vi "CSM - Read INI String.vi"(4 "Write If not found?(F)":bool, 5 "Section Name(\"\" as Default)":string, 7 "error in (no error)":errorcluster, 8 ">> Default Value >>":string, 9 "String in":string) -> (1 "error out":errorcluster, 2 "Key Found?":bool, 3 "String out":string)   [LabVIEW 2017, in "INI-Static-Variable-Support.lvlib"]
uses:
  INI-Static-Variable-Support.lvlib
  _fgv-oper.ctl
  global-csm-ini-db-change-flag.vi
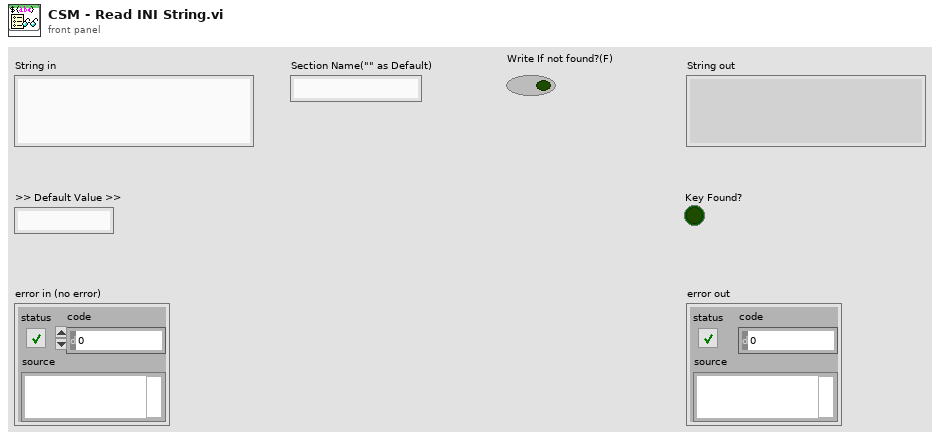
[diagram p1: front panel]
types:
  T1 = typedef "INI-Static-Variable-Support.lvlib/_fgv-oper.ctl" = enum16{"Read", "Write", "Sync", "Sessions", "List Keys", "Load", "List Files", "List Variables", "List Permanent Variables", "Mark Temp Variable as Permenent", "unload", "INIConfig(Memory)", "Reset", "Restore Variable Value"}
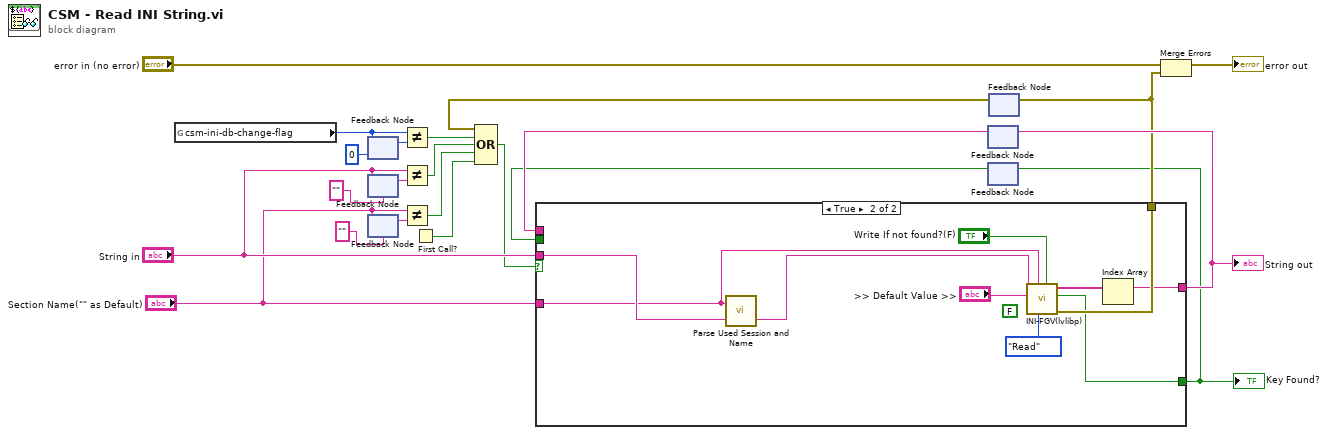
[diagram p0: block diagram]
diagram:
  n1 = global read "global-csm-ini-db-change-flag.vi" "csm-ini-db-change-flag"() -> (w20:u64)
  n2 = feedback #1(u64 0 ("csm-ini-db-change-flag")) -> (w19:u64)
  n3 = feedback-in #1(w20) -> ()
  n4 = feedback #2("") -> (w17:string)
  n5 = feedback-in #2("String in") -> ()
  n6 = feedback #3("") -> (w16:string)
  n7 = feedback-in #3("Section Name(\"\" as Default)") -> ()
  n8 = Not Equal?(x=w20, y=w19) -> (x != y?=w18:bool)
  n9 = Not Equal?(x="String in", y=w17) -> (x != y?=w13:bool)
  n10 = Not Equal?(x="Section Name(\"\" as Default)", y=w16) -> (x != y?=w12:bool)
  n11 = First Call?() -> (First Call?: T/F=w1:bool)
  n12 = feedback #4() -> (w10:string)  [unwired: 1 in]
  n13 = feedback #5() -> (w7:bool)  [unwired: 1 in]
  n14 = feedback #6() -> (w6:errorcluster)  [unwired: 1 in]
  n15 = Compound Arithmetic op=OR(w6, w18, w13, w12, w1) -> (w5:bool)
  n16 = case shown="True" w5 {
    tunnel: [_ w32] -> w9
    tunnel: [w24 w29] -> w11
    tunnel: [w23 w30] -> w8
    tunnel: "String in" -> [_ w27]
    tunnel: "Section Name(\"\" as Default)" -> [_ w25]
    tunnel: w10 -> [w24 _]
    tunnel: w7 -> [w23 _]
    frame False {
    }
    frame True {
      (unwired) FALSE ("Raw String? (F)")
      n17 = call "Parse Used Session and Name.vi"("name"=w27, "Section Name(\"\" as Default)"=w25) -> ("used name"=w26:string)  [unwired: 1 in]
      n18 = call "INI-FGV(lvlibp).vi"("Write If not found?"="Write If not found?(F)", "Enum"=_fgv-oper."Read", "Prefered Section"=w25, ">> Default Value >>"=">> Default Value >>", ">> Variable Name >>"=w26) -> ("error out"=w32:errorcluster, "Key?"=w30:bool, "Array"=w31:string[])  [unwired: 3 in, 1 out]
      n19 = Index Array(array=w31) -> (element=w29:string)  [unwired: 1 in]
    }
  }
  "String out" <- w11
  "Key Found?" <- w8
  n20 = feedback-in #4(w11) -> ()
  n21 = feedback-in #5(w8) -> ()
  n22 = feedback-in #6(w9) -> ()
  n23 = Merge Errors("error in (no error)", w9) -> (→"error out":errorcluster)
